vi "parse_camera_data_representation.vi"(2 "String":string="U16", 3 "Def Camera":refnum<class "Camera.lvclass">) -> (0 "error out":errorcluster, 1 "Data Representation Out":enum16{"U8", "I8", "U16", "I16"}(ring)=enum."U16")   [LabVIEW 2017]
uses:
  classes/HardwareObjects/Camera/Camera.lvclass
  classes/HardwareObjects/Camera/Camera.lvclass/Camera.ctl
  classes/HardwareObjects/Camera/Read Data Representation.vi
  <vilib>/Utility/error.llb/Error Cluster From Error Code.vi
  <vilib>/ErrorRing/Error Ring.xnode
panel:
  out "Data Representation":enum16{"U8", "I8", "U16", "I16"}(ring)=enum."U16"
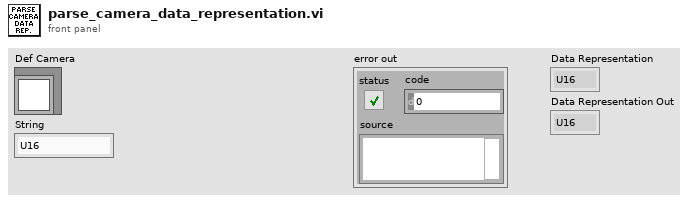
[diagram p1: front panel]
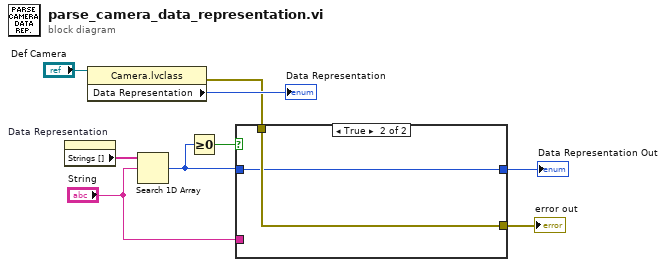
[diagram p0: block diagram]
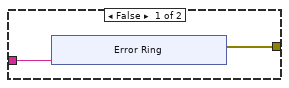
[diagram p2: hidden frame]
diagram:
  n1 = property on="Data Representation" class="Enum (strict)"() -> ("Strings []"=w7:string[])  [unwired: 2 in, 2 out]
  n2 = property class="Camera.lvclass"(reference="Def Camera") -> (error out=w1:errorcluster, "Data Representation"=→"Data Representation":enum16{"U8", "I8", "U16", "I16"})  [unwired: 1 in, 1 out]
  n3 = Search 1D Array(1D array=w7, element="String") -> (index of element=w3:i32)  [unwired: 1 in]
  n4 = Greater Or Equal To 0?(x=w3) -> (x >= 0?=w6:bool)
  n5 = case shown="True" w6 {
    tunnel: w3 -> [_ w19]
    tunnel: "String" -> [w10 _]
    tunnel: [w11 w20] -> w4
    tunnel: [_ w19] -> w2
    tunnel: w1 -> [_ w20]
    frame False {
      n6 = xnode "Error Ring"("parameter 0"=w10) -> ("error out"=w11:errorcluster)
    }
    frame True {
    }
  }
  "error out" <- w4
  "Data Representation Out" <- w2
